vi "2 Shift Goal.vi"   [LabVIEW 2011]
doc: "Uses the values for current and drift to determine how much the boat should point off of it's target. Adds this to the current waypoints location and returns it."
uses:
  2 Typedefs/UTM Circle.ctl
  2 Classes/Waypoint/Waypoint.lvclass
  2 Globals/2 Global.vi
types:
  T1 = typedef "UTM Circle.ctl" = cluster{"UTM Zone":dbl, "Hemisphere":enum16{"North", "South"}, "East":dbl, "North":dbl, "Radius":dbl}
  T2 = typedef "UTM Location.ctl" = cluster{"UTM Zone":i32, "Hemisphere":enum16{"North", "South"}, "East":dbl, "North":dbl}
  T3 = typedef "Velocity.ctl" = cluster{"East":dbl, "North":dbl}
  T4 = typedef "heading.ctl" = dbl
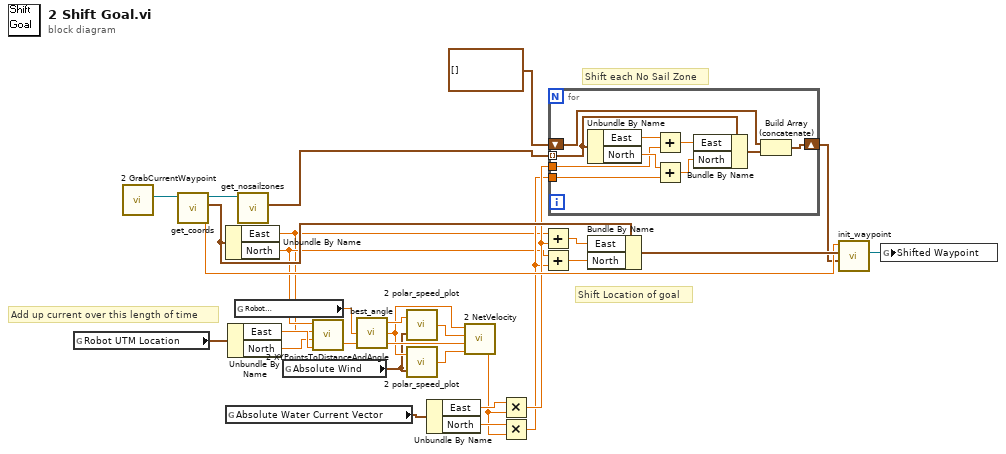
[diagram p0: block diagram]
diagram:
  # "Shift Location of goal"
  # "Add up current over this length of time"
  # "Shift each No Sail Zone"
  n1 = global read "2 Global.vi" "Robot UTM Location"() -> (w6:T2)
  n2 = call "2 GrabCurrentWaypoint.vi"() -> ("Current Waypoint"=w1:refnum<class "Waypoint.lvclass">)  [unwired: 11 in]
  n3 = call-dynamic "get_coords.vi"("Waypoint in"=w1) -> ("Tolerance (meters?)"=w14:dbl, "Coords"=w30:T2, "Waypoint out"=w16:refnum<class "Waypoint.lvclass">)  [unwired: 7 in, 1 out]
  n4 = Unbundle By Name(w30) -> ("East"=w2:dbl, "North"=w3:dbl)
  n5 = global read "2 Global.vi" "Absolute Water Current Vector"() -> (w29:T3)
  n6 = Unbundle By Name(w6) -> ("East"=w5:dbl, "North"=w4:dbl)
  n7 = global read "2 Global.vi" "Robot\nHeading"() -> (w8:T4)
  n8 = call-dynamic "get_nosailzones.vi"("Waypoint in"=w16) -> ("No Sail Circles"=w13:T1[])  [unwired: 7 in, 2 out]
  n9 = global read "2 Global.vi" "Absolute Wind"() -> (w18:T3)
  n10 = call "2 XYPointsToDistanceAndAngle.vi"("East 2"=w5, "North 2"=w4, "East 1"=w2, "North 1"=w3) -> ("Angle Diff"=w7:dbl)  [unwired: 1 out]
  n11 = call "best_angle.vi"("Waypoint Heading"=w7, "Current Heading"=w8) -> ("Heading Candidate 2"=w23:dbl, "Heading Candidate 1"=w19:dbl, "Best Angle"=w20:dbl)  [unwired: 1 in]
  n12 = call "2 polar_speed_plot.vi"("Wind Vector"=w18, "Boat Angle"=w20) -> ("Velocity"=w22:dbl)
  n13 = call "2 polar_speed_plot.vi"("Wind Vector"=w18, "Boat Angle"=w19) -> ("Velocity"=w21:dbl)
  n14 = Unbundle By Name(w29) -> ("East"=w26:dbl, "North"=w25:dbl)
  n15 = call "2 NetVelocity.vi"("Speed 2"=w21, "Angle 2"=w23, "Speed 1"=w22, "Angle 1"=w19) -> ("Net Velocity"=w24:dbl)  [unwired: 7 in]
  n16 = Multiply(x=w26, y=w24) -> (x*y=w12:dbl)
  n17 = Multiply(x=w25, y=w24) -> (x*y=w11:dbl)
  n18 = Add(x=w2, y=w12) -> (x+y=w28:dbl)
  n19 = Add(x=w3, y=w11) -> (x+y=w27:dbl)
  n20 = for {
    tunnel: w13 -> [w39] mode=indexing
    tunnel: w12 -> [w32]
    tunnel: w11 -> [w31]
    shift-right: [w37] -> w9
    shift-left: T1[] [] -> [w40]
    n21 = Unbundle By Name(w39) -> ("East"=w34:dbl, "North"=w33:dbl)
    n22 = Add(x=w34, y=w32) -> (x+y=w35:dbl)
    n23 = Add(x=w33, y=w31) -> (x+y=w36:dbl)
    n24 = Bundle By Name(cluster=w39, "East"=w35, "North"=w36) -> (w38:T1)
    n25 = Build Array (concatenate)(w40, w38) -> (w37:T1[])
  }
  n26 = Bundle By Name(cluster=w30, "East"=w28, "North"=w27) -> (w17:T2)
  n27 = call "init_waypoint.vi"("No Sail Circles"=w9, "Coords"=w17, "Tolerance (m)"=w14) -> ("Waypoint Out"=w15:refnum<class "Waypoint.lvclass">)  [unwired: 8 in]
  n28 = global write "2 Global.vi" "Shifted Waypoint"(w15) -> ()
